vi "GUI_Bella_Control_Center_iP2.vi"() -> ()   [LabVIEW 2020]
uses:
  Shared/GUI_Template/GUI_master/tcp_new_data_event.ctl
  Shared/GUI_Template/GUI_master/tcp new data cluster.ctl
  GUI_TestStand/Fire button.ctl
  Device Drivers/DG645/subVIs/TriggerSource_TypDef.ctl
  <vilib>/Utility/config.llb/Write Key (I32).vi
  <vilib>/Platform/browser.llb/Open URL in Default Browser (string).vi
  <vilib>/Utility/config.llb/NI_LVConfig.lvlib
panel:
  in  "DPM intercept":dbl=94.0 format="%#_13g"
  in  "DPM Direction 3":bool=TRUE
  in  "Move SMF":bool=TRUE
  in  "DPM Direction":bool=TRUE
  in  "Move DPM":bool=TRUE
  in  "Position.Ch3::19":dbl caption="Target Microscope Z" min=0.0 max=100.0 format="%.3f"
  in  "GUIdevice 19":string="MCD-PL1-NewmarkDPMXZ"
  in  "Position.Axis 3::18":dbl caption="ESP6 focal spot mirror" min=0.0 max=100.0 format="%.3f"
  in  "Position.Axis 3::16":dbl caption="ESP5 Target Lateral" min=-200.0 max=200.0 format="%.3f"
  in  "Position.Axis 1::16":dbl caption="ESP5 Target Focus" min=-200.0 max=200.0 format="%.3f"
  in  "GUIdevice 18":string="MCD-PL1-NewmarkDPMXZ"
  in  "GUIdevice 16":string="MCD-PL1-NewmarkDPMXZ"
  in  "Position.Axis 1::14":dbl caption="Debris Shield" min=0.0 max=200.0 format="%.3f"
  in  "Position.Stage B::12":dbl caption="DPM Y" min=-100.0 max=105.0 format="%.3f"
  in  "Position.Stage C::11":dbl caption="DPM Z" min=-100.0 max=100.0 format="%.3f"
  in  "GUIdevice 14":string="MCD-PL1-NewmarkDPMXZ"
  in  "GUIdevice 12":string="MCD-PL1-NewmarkDPMXZ"
  in  "Position.Stage A::11":dbl caption="DPM X" min=-400.0 max=400.0 format="%.3f"
  in  "GUIdevice 11":string="MCD-PL1-NewmarkDPMXZ"
  out "got manpar ofi bool data":bool
  out "got manpar ofi data":bool
  out "set expt editor":bool
  in  "Delay.Ch D::10":dbl=-1.631e-06 caption="Delay D" min=-0.1 max=20.0 format="%.4f"
  in  "value6::42":dbl=0.006 caption="PostScanRate" min=0.1 max=1.0 format="%#_3f"
  in  "value5::42":dbl=0.006 caption="1BL-2BL-\nSplitter-Rpcnt" min=-9999999.0 max=9999999.0 format="%#_6p"
  in  "value6::43":bool=TRUE caption="GhostFoil-In"
  in  "value5::43":bool=TRUE caption="1BL-Energy\nMeter-In"
  in  "value4::43":bool=TRUE caption="2BLFoil-In"
  in  "value3::43":bool=TRUE caption="1BLFoil-In"
  in  "value2::43":bool=TRUE caption="ClunkerIn"
  out "CurrentStatus":string
  in  "MoveStage":bool
  in  "Position.Ch1::44":dbl caption="Current Position" min=0.0 max=150.0
  in  "GUIdevice 44":string="STAGE-LT-Megattenuator"
  in  "GUIdevice 43":string="MANPAR-BELLA-OFI-Boolean"
  in  "GUIdevice 42":string="MANPAR-BELLA-OFI"
  out "HPD2 to match HPD":dbl
  in  "Save \ncreenshots":bool
  out "error out":errorcluster
  out "HPD - focus":dbl
  in  "value1::42":dbl=230.0 caption="focus on HPD" min=-9999999.0 max=9999999.0
  in  "value0::43":bool=TRUE caption="SCS"
  in  "Thales.DIAG_CU_Output_Percent_1::37":dbl caption="Amp2 att (%)" min=1.0 max=100.0 step=500.0 format="%.2f"
  in  "GUIdevice 37":string="SVE-LT-Thales"
  in  "Scan":T1(ring)
  in  "LogTable":bool
  in  "New Google\nExpLog for new day?":bool=TRUE
  out "standard output":string
  in  "Create Log":bool caption="LogTable"
  in  "Position.Channel 5::31":T2(ring) caption="FROG foil"
  in  "Position.Channel 2::31":T2(ring) caption="Little Rick"
  in  "Step size 2":dbl=20.0 caption="Step size" min=-22.0 max=22.0
  in  "Position.Axis 4::33":dbl caption="Holy M V F4" min=-100000.0 max=100000.0 step=500.0
  in  "Position.Axis 3::33":dbl caption="Holy M H F3" min=-1000000.0 max=1000000.0 step=500.0
  in  "Position.Axis 2::33":dbl caption="Bessel M3 V F2" min=-100000.0 max=100000.0 step=500.0
  in  "Position.Axis 1::33":dbl caption="Bessel M3 H F1" min=-100000.0 max=100000.0 step=500.0
  in  "GUIdevice 33":string="MCD-PL1-picosOFI1"
  in  "GUIdevice 4":string="STAGE-PL1-Capstage1"
  in  "GUIdevice 31":string="1WIRE-BELLA-Flipper"
  in  "Amplitude.Ch GH::10":dbl=-1.631e-06 caption="Shot Shutter V" min=0.5 max=5.0 format="%.1f"
  in  "Rate (Hz)":dbl=0.3
  in  "Heater Alignment Directions":bool
  in  "Position.Axis 3::15":dbl caption="XY" min=-3.0 max=16.0 format="%.4f"
  in  "Position.Axis 2::15":dbl caption="Y" min=-3.0 max=17.0 format="%.4f"
  in  "Position.Axis 1::15":dbl caption="X" min=-3.0 max=13.0 format="%.4f"
  in  "GUIdevice 24":string="STAGE-HEAT-TL1"
  in  "Encoder position::23":dbl caption="position HPD2" min=0.0 max=600.0 format="%.1f"
  in  "position::3":dbl caption="position HPD" min=0.0 max=600.0 format="%.1f"
  in  "GUIdevice 23":string="STAGE-HPD-Far"
  in  "GUIdevice 22":string="MANPAR-BELLA-FireCont"
  in  "Allow Fire Continues":bool
  out "Fire continues Indicator":bool caption="firing"
  in  "Fire Button":T3=TRUE
  in  "Trigger.Source::10":T4 caption="SRS Trigger Mode"
  out "Absolute discharge timing":dbl caption="delay from pk" format="%#.3p"
  in  "Delay.Ch E::17":dbl caption="Timing box" min=-0.1 max=0.1 format="%.3p"
  in  "value0::22":bool caption="Fire continuosly"
  in  "GUIdevice 15":string="MCD-HEAT-ESP1"
  in  "GUIdevice 17":string="DDG-AA-SRS0"
  out "error IO 2":errorcluster
  out "tcp data event":T5
  in  "UDP error message":string
  in  "GUIdevice 13":string="DDG-AA-SRS2"
  in  "GUIdevice 2":string="MANPAR-BELLA-General"
  in  "GUIdevice 10":string="DDG-AA-ShotCntrl"
  in  "GUIdevice 1":string="HEX-PL1-1"
  in  "GUIdevice 3":string="STAGE-HPD-Tel"
  in  "Position.Axis 1::9":dbl caption="Comp1 Translation" min=-50.0 max=50.0 format="%.3f"
  in  "GUIdevice 9":string="STAGE-1BL-Compression"
  in  "stop":bool
  # "BELLA ip2 CONTROL CENTER"
  # "Scan"
  # "Safety"
  # "needs manpar-bella-ofi on\nMANPAR-BELLA-OFI-Boolean"
  # "Discharge timing (s)"
  # "1wire"
  # "DG"
  # "PICOS"
  # "Heater timing (s)"
  # "HPD Stage"
  # "Megattenuator Stage"
  # "Attenuate"
  # "OUT"
  # "IN"
  # "Compressor"
  # "Heater Alignment"
  # "Heat ESP0"
  # "Heat ESP1"
  # "Heat Pico"
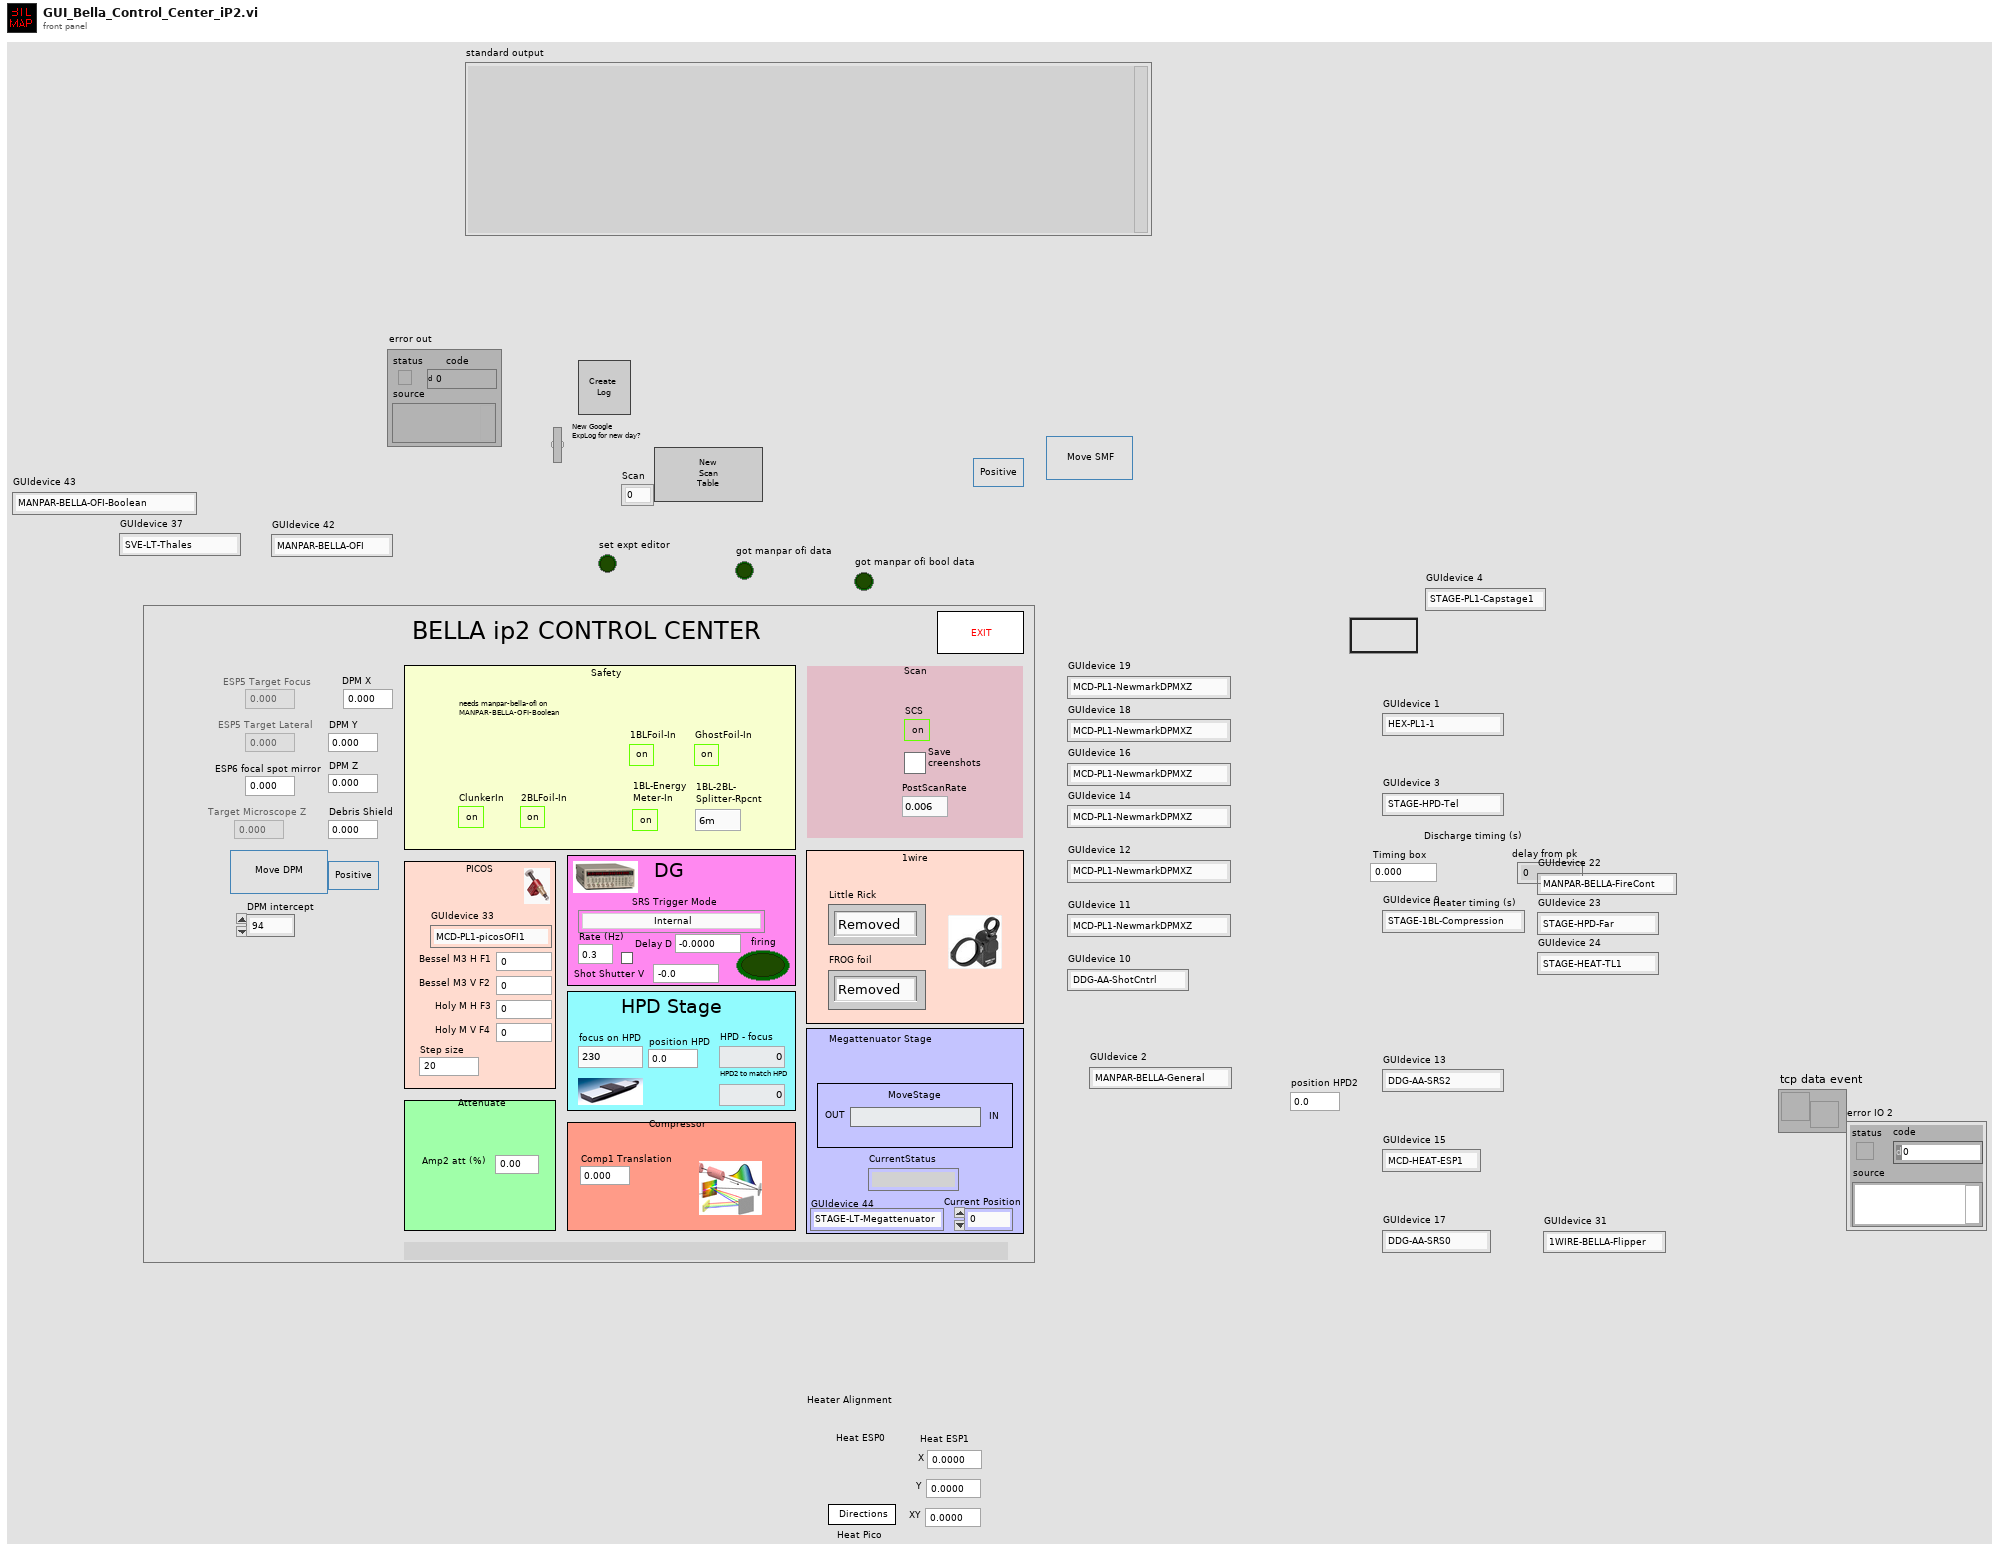
[diagram p1: front panel]
types:
  T1 = enum16{"0", "1", "2", "3", "4", "5", "6", "7", "8", "9", "10", "11", "12", "13", "14", "15", "16", "17", "18", "19", "20", "21", "22", "23", "24", "25", "26", "27", "28", "29", "30", "31", "32", "33", "34", "35", "36", "37", "38", "39", "40", "41", "42", "43", "44", "45", "46", "47", "48", "49", "50", "51", "52", "53", "54", "55", "56", "57", "58", "59", "60", "61", "62", "63", "64", "65", "66", "67", "68", "69", "70", "71", "72", "73", "74", "75", "76", "77", "78", "79", "81", "82", "83", "84", "85", "86", "87", "88", "89", "90", "91", "92", "93", "94", "95", "96", "97", "98", "99", ""}
  T2 = enum16{"Removed", "Inserted", "Unknown", "Moving"}
  T3 = typedef "Fire button.ctl" = bool
  T4 = typedef "TriggerSource_TypDef.ctl" = enum16{"Internal", "External rising edges", "External falling edges", "Single shot external rising edges", "Single shot external falling edges", "Single shot", "Line"}
  T5 = typedef "tcp_new_data_event.ctl" = refnum<user-event>
  T6 = typedef "tcp new data cluster.ctl" = cluster{"EventEnum":enum16{"new data", "connection status update"}, "Device name":string}
  T7 = enum8{"Enabled", "Disabled", "Disabled and Grayed Out"}
  T8 = enum32{"invalid app kind", "Development System", "Run Time System", "Student Edition", "Embedded LabVIEW", "Evaluation", "Custom"}
  T9 = enum32{"Invalid", "Standard", "Closed", "Hidden", "Minimized", "Maximized"}
  T10 = typedef "imagedata.ctl" = cluster{"image type":i32, "image depth":i32, "image":u8[], "mask":u8[], "colors":u32[], "Rectangle":cluster{"left":i16, "top":i16, "right":i16, "bottom":i16}}
  T11 = typedef "NI_LVConfig.lvlib/Config Data RefNum.ctl" = refnum<k1>
  T12 = cluster{"Core":cluster{"Current VI Reference":refnum<vi>, "Close Panel on Exit?":bool}, "Heater timing offset":dbl, "Discharge timing offset":dbl, "Jet trigger":bool, "Tik1":u32, "Tik2":u32, "Fire Continues Allowed":bool}
  T13 = cluster{"Current VI Reference":refnum<vi>, "Close Panel on Exit?":bool}
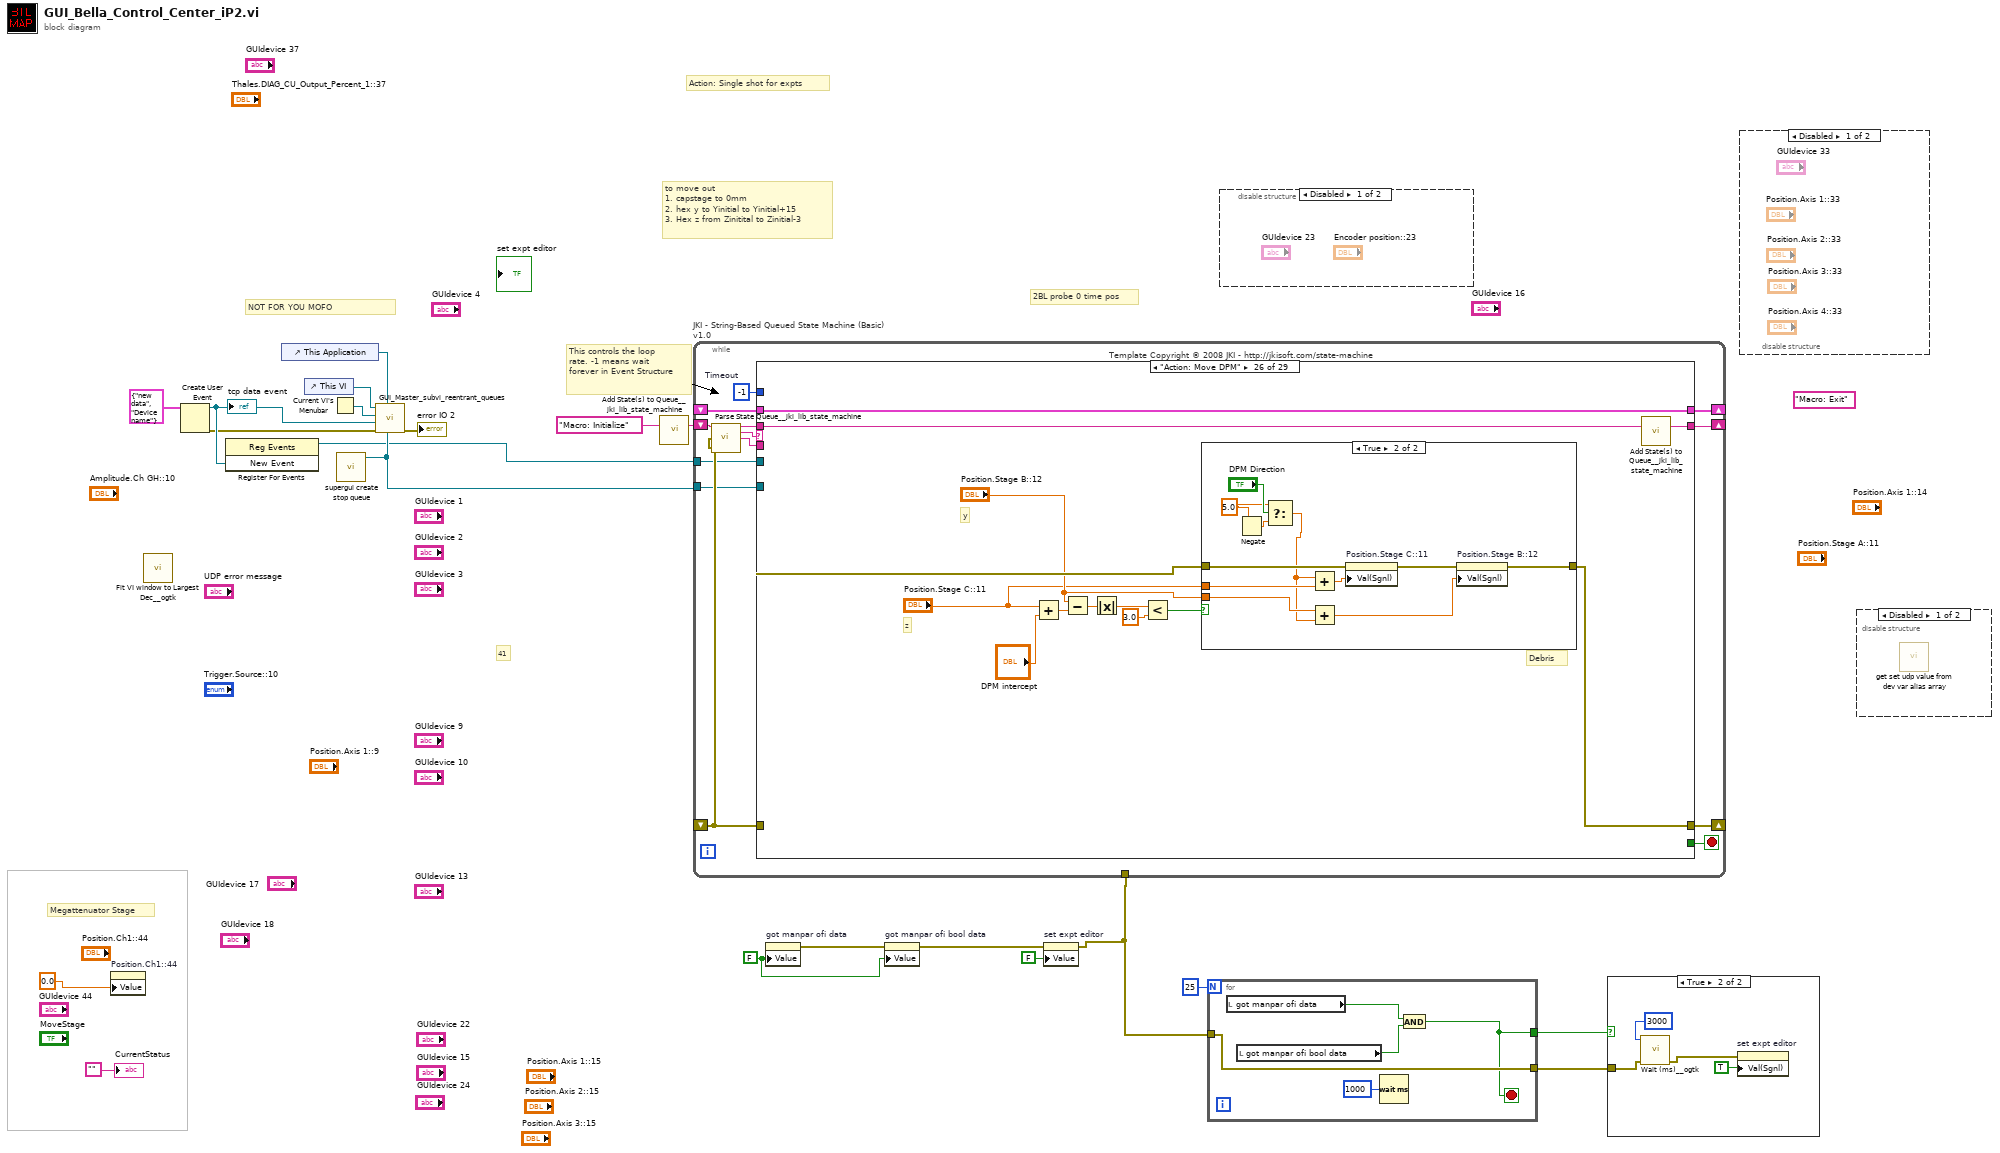
[diagram p0: block diagram]
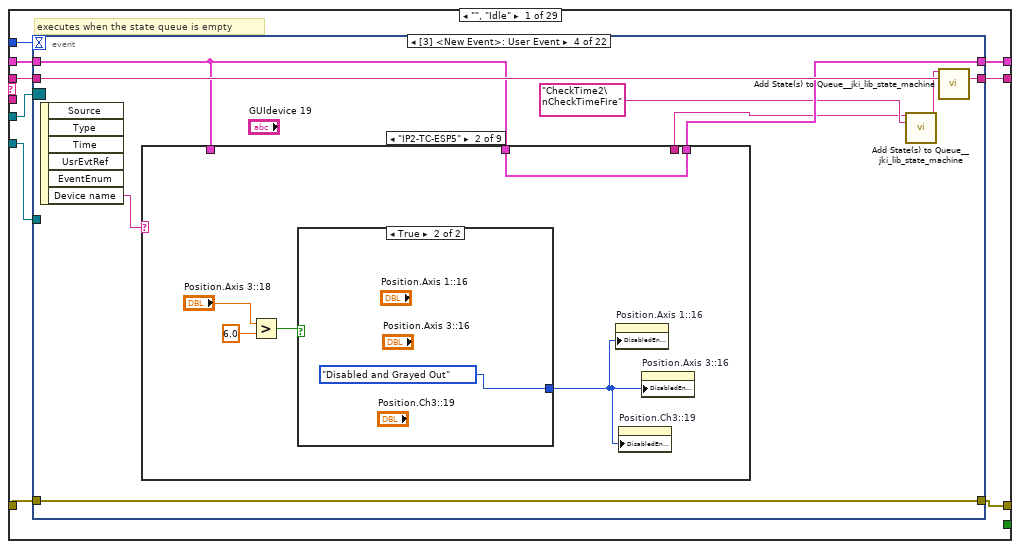
[diagram p6: hidden frame]
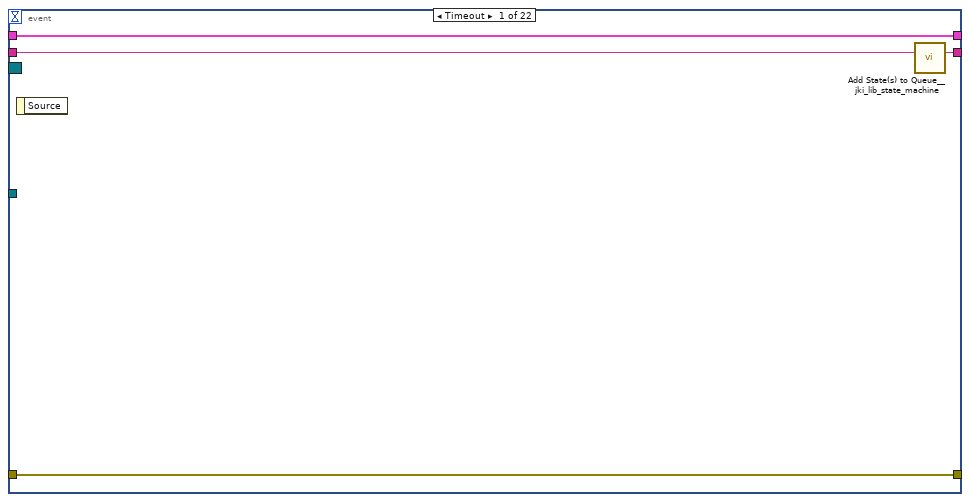
[diagram p7: hidden frame]
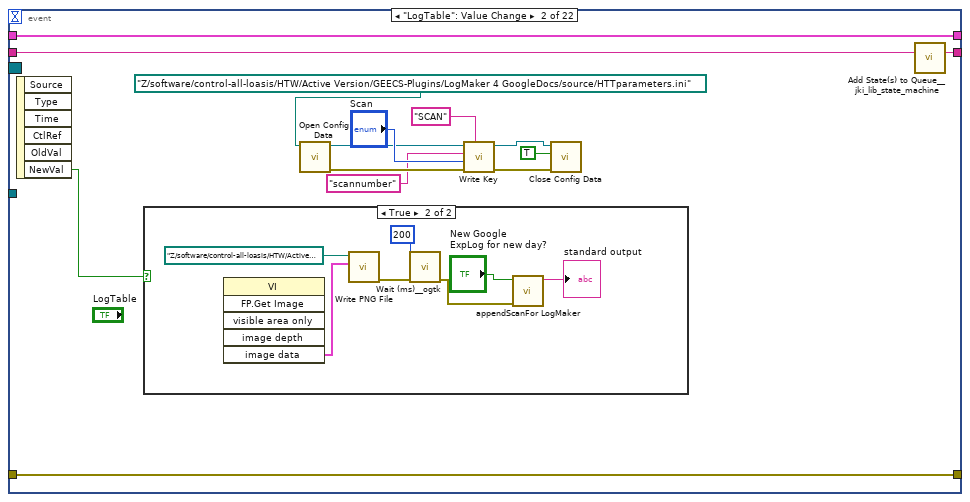
[diagram p8: hidden frame]
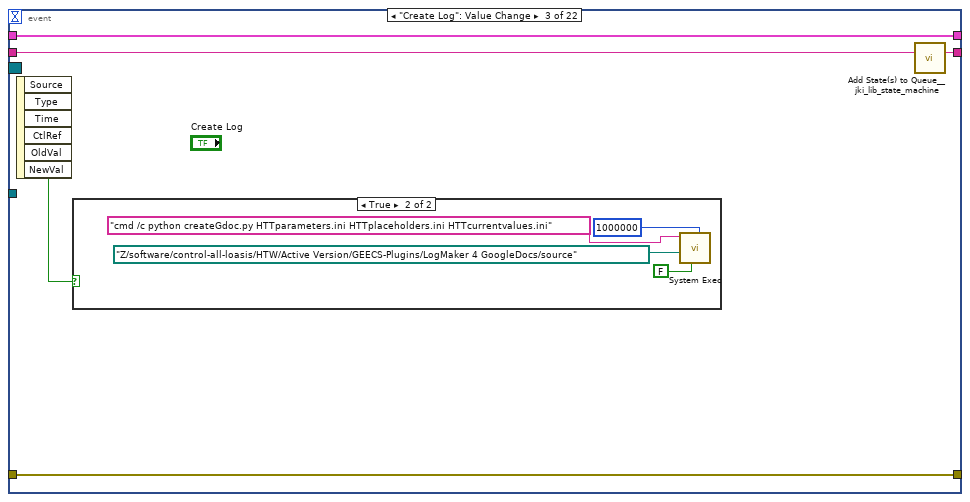
[diagram p10: hidden frame]
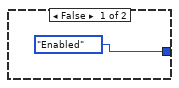
[diagram p13: hidden frame]
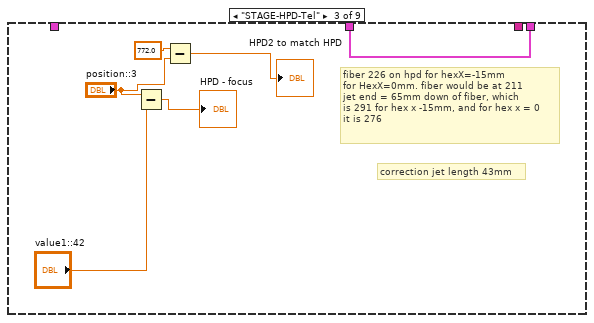
[diagram p14: hidden frame]
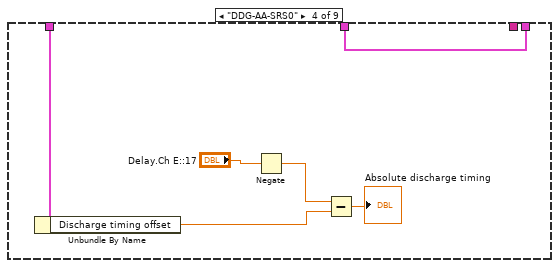
[diagram p15: hidden frame]
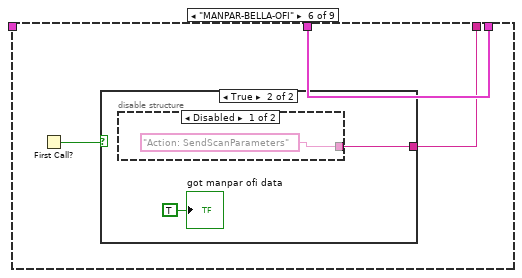
[diagram p17: hidden frame]
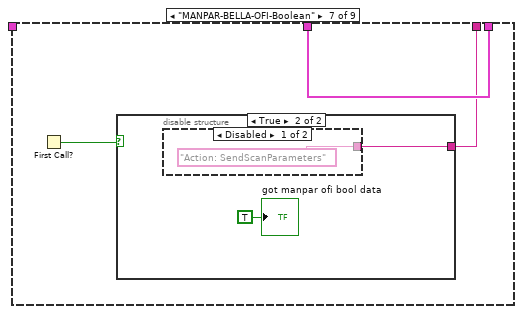
[diagram p20: hidden frame]
diagram:
  w5 = FALSE ("got manpar ofi data")
  (unwired) "Macro: Exit"
  # "41"
  # "Megattenuator Stage"
  # "2BL probe 0 time pos"
  # "Action: Single shot for expts"
  # "to move out\n1. capstage to 0mm\n2. hex y to Yinitial to Yinitial+15\n3. Hex z from Zinitital to Zinitial-3"
  # "This controls the loop rate. -1 means wait forever in Event Structure"
  # "NOT FOR YOU MOFO"
  n1 = property on="Position.Ch1::44" class="DigNum (strict)"("Value"=0.0 ("Position.Ch1::44")) -> ()  [unwired: 2 in, 2 out]
  n2 = call <userlib>:"Fit VI window to Largest Dec__ogtk.vi"() -> ()  [unwired: 6 in, 2 out]
  n3 = Create User Event(user event datatype=T6 {"EventEnum"=enum."new data", "Device name"="Device name"} ("New Event")) -> (user event=w20:refnum<user-event>, error out=w19:errorcluster)  [unwired: 1 in]
  "tcp data event" <- w20
  n4 = register-events(w20) -> (reference out=w11:refnum<event-registration>)  [unwired: 2 in, 1 out]
  n5 = control-ref of="This Application"() -> (w21:refnum<vi>)
  n6 = control-ref of="This VI"() -> (w15:refnum<vi>)
  n7 = Current VI's Menubar() -> (w17:refnum<k9>)
  n8 = call "supergui create stop queue.vi"() -> ("STOP Queue out"=w12:refnum<queue>)  [unwired: 11 in]
  n9 = call "GUI_Master_subvi_reentrant_queues.vi"("STOP Queue in"=w12, "This Application"=w21, "error in (no error)"=w19, "tcp data event"=w20, "Caller menu reference"=w17, "Caller VI ref"=w15) -> ("error out"=→"error IO 2":errorcluster)  [unwired: 5 in]
  n10 = call <vilib>:"Add State(s) to Queue__jki_lib_state_machine.vi"("State(s) in (\"\")"="Macro: Initialize") -> ("States Out"=w13:string)  [unwired: 14 in]
  n11 = property on="got manpar ofi data" class="Bool (strict)"("Value"=w5) -> (error out=w6:errorcluster)  [unwired: 2 in, 1 out]
  n12 = property on="got manpar ofi bool data" class="Bool (strict)"(error in=w6, "Value"=w5) -> (error out=w7:errorcluster)  [unwired: 1 in, 1 out]
  n13 = property on="set expt editor" class="Bool (strict)"(error in=w7, "Value"=FALSE ("set expt editor")) -> (error out=w4:errorcluster)  [unwired: 1 in, 1 out]
  n14 = while "JKI - String-Based Queued State Machine (Basic) v1.0" {
    shift-right: [w27] -> _
    shift-left: _ -> [w26]
    shift-right: [w30] -> _
    shift-left: _ -> [w24]
    shift-right: [w29] -> _
    shift-left: w13 -> [w31]
    tunnel: w11 -> [w23]
    tunnel: w12 -> [w22]
    tunnel: w4 -> [_]
    stop <- w28 stop-if-true
    w25 = -1  # Timeout
    # "Template Copyright © 2008 JKI - http://jkisoft.com/state-machine"
    n15 = call <vilib>:"Parse State Queue__jki_lib_state_machine.vi"("State Queue"=w31, "Error In (no error)"=w24) -> ("Remaining States"=w33:string, "Current State"=w34:string, "Arguments"=w32:string)  [unwired: 11 in]
    n16 = case shown="\"Action: Move DPM\"" w34 {
      selector: w34 -> [_ _ w296 _ _ _ _ _ _ _ _ _ _ _ _ _ _ _ _ _ _ _ _ _ _ _ _ _ _]
      tunnel: w33 -> [w43 w295 w300 w318 w324 w329 w333 w344 w350 w354 w358 w364 w375 w401 w406 w419 w423 w429 w438 w475 w486 w498 w510 w517 w521 w534 w550 w558 w565]
      tunnel: w32 -> [_ _ _ _ _ _ _ _ _ _ _ w359 w369 _ _ _ _ _ _ _ _ _ _ _ _ _ _ _ _]
      tunnel: w26 -> [w41 w292 w298 w309 w321 w327 w330 _ w345 w351 w356 w362 w371 w398 w403 w416 w420 w426 w435 w463 w482 w492 w507 w515 w519 w532 w547 w555 w562]
      tunnel: [w40 w293 w302 w315 errorcluster {"status"=FALSE, "code"=0, "source"=""} ("error out") w326 w331 w341 w346 w352 w355 w360 w372 w399 w404 w417 w421 w427 w436 w473 w480 w487 w508 w514 w518 w524 w548 w556 w563] -> w30
      tunnel: w24 -> [w39 w293 w301 w315 w320 w326 w331 w341 w347 w352 w355 w361 w373 w399 w404 w417 w421 w427 w436 w473 w484 w488 w508 w514 w518 w525 w548 w556 w563]
      tunnel: [w42 w294 w299 w317 w323 w328 w332 w343 w349 w353 w357 w363 w374 w400 w405 w418 w422 w428 w437 w474 w485 w497 w509 w516 w520 w533 w549 w557 w564] -> w29
      tunnel: [_ _ _ _ _ TRUE _ _ _ _ _ _ _ _ _ _ _ _ _ _ _ _ _ _ _ _ _ _ _] -> w28
      tunnel: [w35 w292 w298 w316 w321 w327 w330 w342 w345 w351 w356 w362 w371 w398 w403 w416 w420 w426 w435 w472 w482 w491 w506 w515 w519 w532 w547 w555 w562] -> w27
      tunnel: w25 -> [w38 _ _ _ _ _ _ _ _ _ _ _ _ _ _ _ _ _ _ _ _ _ _ _ _ _ _ _ _]
      tunnel: w23 -> [w37 _ _ _ _ _ _ _ _ _ _ _ _ _ _ _ _ _ _ _ _ _ _ _ _ _ _ _ _]
      tunnel: w22 -> [w36 _ _ _ _ _ _ _ _ _ _ _ _ _ _ w408 _ _ _ _ _ _ _ _ _ _ _ _ _]
      frame "", "Idle" {
        # "executes when the state queue is empty"
        n17 = event shown="[3] <New Event>: User Event" {
          selector: w37 -> [_ _ _ _ _ _ _ _ _ _ _ _ _ _ _ _ _ _ _ _ _ _]
          dyn-events: _ -> [_ _ _ _ _ _ _ _ _ _ _ _ _ _ _ _ _ _ _ _ _ _]
          timeout: w38 -> [_ _ _ _ _ _ _ _ _ _ _ _ _ _ _ _ _ _ _ _ _ _]
          tunnel: w43 -> [w47 w61 w73 w86 w129 w131 w136 w141 w146 w156 w166 w176 w186 w196 w205 w213 w222 w246 w256 w263 w265 w291]
          tunnel: [w46 w60 w72 w85 w128 w132 w137 w142 w147 w157 w167 w177 w187 w197 w206 w213 w221 w244 w256 w263 w264 w290] -> w42
          tunnel: w41 -> [w44 w58 w70 w82 w126 w134 w139 w144 w149 w159 w169 w179 w189 w199 w208 w212 w224 w248 w257 w262 w272 w288]
          tunnel: [w45 w59 w71 w84 w127 w133 w138 w143 w148 w158 w168 w178 w188 w198 w207 w210 w227 w247 w255 w261 w271 w289] -> w40
          tunnel: w39 -> [w45 w59 w71 w84 w127 w133 w138 w143 w148 w158 w168 w178 w188 w198 w207 w211 w226 w247 w255 w261 w271 w289]
          tunnel: [w44 w58 w70 w81 w126 w134 w139 w144 w149 w159 w169 w179 w189 w199 w208 w212 w225 w248 w257 w262 w272 w288] -> w35
          tunnel: w36 -> [_ _ _ _ _ _ _ _ _ _ _ _ _ _ _ _ _ _ _ _ _ _]
          event Timeout {
            n18 = event-data() -> ()  [unwired: 1 in, 1 out]
            n19 = call <vilib>:"Add State(s) to Queue__jki_lib_state_machine.vi"("State(s) in (\"\")"=w47) -> ("States Out"=w46:string)  [unwired: 14 in]
          }
          event "LogTable": Value Change {
            n20 = event-data() -> ("NewVal"=w48:bool)  [unwired: 1 in, 5 out]
            n21 = case shown="True" w48 {
              frame False {
              }
              frame True {
                n22 = invoke class="VI" method="FP.Get Image"() -> ("image data"=w68:T10)  [unwired: 6 in, 5 out]
                n23 = call <vilib>:"Write PNG File.vi"("image data"=w68, "path to PNG file"=path "Z:/software/control-all-loasis/HTW/Active Version/GEECS-Plugins/LogMaker 4 GoogleDocs/source/frontpanel.png" ("report file path")) -> ("error out"=w63:errorcluster)  [unwired: 8 in, 1 out]
                n24 = call <userlib>:"Wait (ms)__ogtk.vi"("error in (no error)"=w63, "milliseconds to wait"=u32 200 ("millisecond timer value")) -> ("error out"=w62:errorcluster)  [unwired: 8 in, 1 out]
                n25 = call "appendScanFor LogMaker.vi"("error in (no error)"=w62, "New Google\nExpLog for new day?"="New Google\nExpLog for new day?") -> ("standard output"=→"standard output":string)  [unwired: 9 in]
              }
            }
            n26 = call <vilib>:"Open Config Data.vi"("configuration file path"=path "Z:/software/control-all-loasis/HTW/Active Version/GEECS-Plugins/LogMaker 4 GoogleDocs/source/HTTparameters.ini") -> ("error out"=w55:errorcluster, "refnum"=w53:T11)  [unwired: 8 in, 1 out]
            n27 = call-poly <vilib>:"Write Key.vi"("section"="SCAN", "error in (no error)"=w55, "value"="Scan", "key"="scannumber", "refnum"=w53) -> ("error out"=w56:errorcluster, "refnum out"=w54:T11)  [unwired: 4 in, 1 out]
            n28 = call <vilib>:"Close Config Data.vi"("error in (no error)"=w56, "write file if changed (T)"=TRUE, "refnum"=w54) -> ()  [unwired: 7 in, 2 out]
            n29 = call <vilib>:"Add State(s) to Queue__jki_lib_state_machine.vi"("State(s) in (\"\")"=w61) -> ("States Out"=w60:string)  [unwired: 14 in]
          }
          event "Create Log": Value Change {
            n30 = event-data() -> ("NewVal"=w69:bool)  [unwired: 1 in, 5 out]
            n31 = case shown="True" w69 {
              frame False {
              }
              frame True {
                n32 = call <vilib>:"System Exec.vi"("expected output size  (4096)"=u32 1000000, "run minimized? (F)"=FALSE, "working directory"=path "Z:/software/control-all-loasis/HTW/Active Version/GEECS-Plugins/LogMaker 4 GoogleDocs/source", "command line"="cmd /c python createGdoc.py HTTparameters.ini HTTplaceholders.ini HTTcurrentvalues.ini") -> ()  [unwired: 4 in, 4 out]
              }
            }
            n33 = call <vilib>:"Add State(s) to Queue__jki_lib_state_machine.vi"("State(s) in (\"\")"=w73) -> ("States Out"=w72:string)  [unwired: 14 in]
          }
          event User Event {
            n34 = event-data() -> ("Device name"=w83:string)  [unwired: 1 in, 5 out]
            n35 = case shown="\"IP2-TC-ESP5\"" w83 {
              tunnel: w82 -> [_ _ _ w103 _ _ _ _ _]
              tunnel: w82 -> [w87 w92 w100 w101 w107 w110 w116 w123 w124]
              tunnel: [w87 w92 w100 w101 w107 w110 w116 w123 w124] -> w81
              tunnel: [_ _ _ _ _ w109 w115 "Check Megattenuator Stage Status" ("State(s) in Front (\"\")") _] -> w78
              frame "False", Default {
              }
              frame "IP2-TC-ESP5" {
                n36 = Greater?(x="Position.Axis 3::18", y=6.0) -> (0:w89:bool)
                n37 = case shown="True" w89 {
                  tunnel: [T7."Enabled" ("Disabled") T7."Disabled and Grayed Out" ("Disabled")] -> w88
                  frame False {
                  }
                  frame True {
                  }
                }
                n38 = property on="Position.Axis 1::16" class="DigNum (strict)"("DisabledEnum"=w88) -> ()  [unwired: 2 in, 2 out]
                n39 = property on="Position.Ch3::19" class="DigNum (strict)"("DisabledEnum"=w88) -> ()  [unwired: 2 in, 2 out]
                n40 = property on="Position.Axis 3::16" class="DigNum (strict)"("DisabledEnum"=w88) -> ()  [unwired: 2 in, 2 out]
              }
              frame "STAGE-HPD-Tel" {
                # "correction jet length 43mm"
                # "fiber 226 on hpd for hexX=-15mm\nfor HexX=0mm. fiber would be at 211\njet end = 65mm down of fiber, which\nis 291 for hex x -15mm, and for hex x = 0\nit is 276"
                n41 = Subtract(x="position::3", y="value1::42") -> (x-y=→"HPD - focus":dbl)
                n42 = Subtract(x=772.0 ("y"), y="position::3") -> (x-y=→"HPD2 to match HPD":dbl)
              }
              frame "DDG-AA-SRS0" {
                n43 = Unbundle By Name(w103) -> ("Discharge timing offset"=w102:dbl)
                n44 = Negate(x="Delay.Ch E::17") -> (-x=w104:dbl)
                n45 = Subtract(x=w104, y=w102) -> (x-y=→"Absolute discharge timing":dbl)
              }
              frame "STAGE-2BL-ProbeDelay" {
              }
              frame "MANPAR-BELLA-OFI" {
                n46 = First Call?() -> (First Call?: T/F=w108:bool)
                n47 = case shown="True" w108 {
                  tunnel: [_ w112] -> w109
                  frame False {
                  }
                  frame True {
                    n48 = disable-structure shown="Disabled" {
                      disable-tunnel: ["Action: SendScanParameters" ("State(s) in Front (\"\")") _] -> w112
                      frame Disabled {
                      }
                      frame Enabled {
                      }
                    }
                    "got manpar ofi data" <- TRUE ("got manpar ofi data")
                  }
                }
              }
              frame "MANPAR-BELLA-OFI-Boolean" {
                n49 = First Call?() -> (First Call?: T/F=w114:bool)
                n50 = case shown="True" w114 {
                  tunnel: [_ w118] -> w115
                  frame False {
                  }
                  frame True {
                    n51 = disable-structure shown="Disabled" {
                      disable-tunnel: ["Action: SendScanParameters" ("State(s) in Front (\"\")") _] -> w118
                      frame Disabled {
                      }
                      frame Enabled {
                      }
                    }
                    "got manpar ofi bool data" <- TRUE ("got manpar ofi bool data")
                  }
                }
              }
              frame "STAGE-LT-Megattenuator" {
                n52 = property on="Position.Ch1::44" class="DigNum (strict)"() -> ("Caption.FontStrike"=w120:bool)  [unwired: 2 in, 2 out]
                n53 = Not(x=w120) -> (.not. x?=w121:bool)
                n54 = property on="MoveStage" class="Bool (strict)"("Visible"=w121) -> ()  [unwired: 2 in, 2 out]
                n55 = property on="CurrentStatus" class="Str"("Visible"=w121) -> ()  [unwired: 2 in, 2 out]
              }
              frame "1WIRE-BELLA-Flipper" {
              }
            }
            n56 = call <vilib>:"Add State(s) to Queue__jki_lib_state_machine.vi"("State(s) in Front (\"\")"=w78, "State(s) in (\"\")"="CheckTime2\nCheckTimeFire" ("State(s) in Front (\"\")")) -> ("States Out"=w79:string)  [unwired: 13 in]
            n57 = call <vilib>:"Add State(s) to Queue__jki_lib_state_machine.vi"("State(s) in Front (\"\")"=w79, "State(s) in (\"\")"=w86) -> ("States Out"=w85:string)  [unwired: 13 in]
          }
          event "stop": Value Change {
            # "Exit Button Value Change (pressed) Event\n(this executes Macro: Exit to terminate the VI)"
            n58 = event-data() -> ()  [unwired: 1 in, 6 out]
            n59 = call <vilib>:"Add State(s) to Queue__jki_lib_state_machine.vi"("State(s) in Front (\"\")"="Macro: Exit", "State(s) in (\"\")"=w129) -> ("States Out"=w128:string)  [unwired: 13 in]
          }
          event Value Change {
            n60 = event-data() -> ()  [unwired: 1 in, 6 out]
            n61 = call <vilib>:"Add State(s) to Queue__jki_lib_state_machine.vi"("State(s) in Front (\"\")"="Action: Fire" ("State(s) in Front (\"\")"), "State(s) in (\"\")"=w131) -> ("States Out"=w132:string)  [unwired: 13 in]
          }
          event "Move DPM": Value Change {
            n62 = event-data() -> ()  [unwired: 1 in, 6 out]
            n63 = call <vilib>:"Add State(s) to Queue__jki_lib_state_machine.vi"("State(s) in Front (\"\")"="Action: Move DPM" ("State(s) in Front (\"\")"), "State(s) in (\"\")"=w136) -> ("States Out"=w137:string)  [unwired: 13 in]
          }
          event "Move SMF": Value Change {
            n64 = event-data() -> ()  [unwired: 1 in, 6 out]
            n65 = call <vilib>:"Add State(s) to Queue__jki_lib_state_machine.vi"("State(s) in Front (\"\")"="Action: Move SMF" ("State(s) in Front (\"\")"), "State(s) in (\"\")"=w141) -> ("States Out"=w142:string)  [unwired: 13 in]
          }
          event "value0::43", "value6::42": Value Change {
            n66 = event-data() -> ()  [unwired: 1 in, 6 out]
            n67 = call <vilib>:"Add State(s) to Queue__jki_lib_state_machine.vi"("State(s) in Front (\"\")"="Action: SendScanParameters" ("State(s) in Front (\"\")"), "State(s) in (\"\")"=w146) -> ("States Out"=w147:string)  [unwired: 13 in]
          }
          event "value2::43": Value Change {
            n68 = event-data() -> ()  [unwired: 1 in, 6 out]
            n69 = local read "GUIdevice 43"() -> (w150:string)
            n70 = Select(t="on", s="value2::43", f="off") -> (s? t:f=w155:string)
            n71 = call "DefaultValue_Variable_MC.vi"("Variable In"="value2", "Default Value"=w155, "Device In"=w150) -> ()  [unwired: 1 in]
            n72 = call <vilib>:"Add State(s) to Queue__jki_lib_state_machine.vi"("State(s) in (\"\")"=w156) -> ("States Out"=w157:string)  [unwired: 14 in]
          }
          event "value3::43": Value Change {
            n73 = event-data() -> ()  [unwired: 1 in, 6 out]
            n74 = local read "GUIdevice 43"() -> (w161:string)
            n75 = Select(t="on", s="value3::43", f="off") -> (s? t:f=w165:string)
            n76 = call "DefaultValue_Variable_MC.vi"("Variable In"="value3", "Default Value"=w165, "Device In"=w161) -> ()  [unwired: 1 in]
            n77 = call <vilib>:"Add State(s) to Queue__jki_lib_state_machine.vi"("State(s) in (\"\")"=w166) -> ("States Out"=w167:string)  [unwired: 14 in]
          }
          event "value4::43": Value Change {
            n78 = event-data() -> ()  [unwired: 1 in, 6 out]
            n79 = local read "GUIdevice 43"() -> (w171:string)
            n80 = Select(t="on", s="value4::43", f="off") -> (s? t:f=w175:string)
            n81 = call "DefaultValue_Variable_MC.vi"("Variable In"="value4", "Default Value"=w175, "Device In"=w171) -> ()  [unwired: 1 in]
            n82 = call <vilib>:"Add State(s) to Queue__jki_lib_state_machine.vi"("State(s) in (\"\")"=w176) -> ("States Out"=w177:string)  [unwired: 14 in]
          }
          event "value5::43": Value Change {
            n83 = event-data() -> ()  [unwired: 1 in, 6 out]
            n84 = local read "GUIdevice 43"() -> (w181:string)
            n85 = Select(t="on", s="value5::43", f="off") -> (s? t:f=w185:string)
            n86 = call "DefaultValue_Variable_MC.vi"("Variable In"="value5", "Default Value"=w185, "Device In"=w181) -> ()  [unwired: 1 in]
            n87 = call <vilib>:"Add State(s) to Queue__jki_lib_state_machine.vi"("State(s) in (\"\")"=w186) -> ("States Out"=w187:string)  [unwired: 14 in]
          }
          event "value6::43": Value Change {
            n88 = event-data() -> ()  [unwired: 1 in, 6 out]
            n89 = local read "GUIdevice 43"() -> (w191:string)
            n90 = Select(t="on", s="value6::43", f="off") -> (s? t:f=w195:string)
            n91 = call "DefaultValue_Variable_MC.vi"("Variable In"="value6", "Default Value"=w195, "Device In"=w191) -> ()  [unwired: 1 in]
            n92 = call <vilib>:"Add State(s) to Queue__jki_lib_state_machine.vi"("State(s) in (\"\")"=w196) -> ("States Out"=w197:string)  [unwired: 14 in]
          }
          event "value5::42": Value Change {
            n93 = event-data() -> ()  [unwired: 1 in, 6 out]
            n94 = Number To Fractional String(number="value5::42", precision (6)=i16 4) -> (F-format string=w201:string)  [unwired: 2 in]
            n95 = call "DefaultValue_Variable_MC.vi"("Variable In"="value5", "Default Value"=w201, "Device In"="GUIdevice 42") -> ()  [unwired: 1 in]
            n96 = call <vilib>:"Add State(s) to Queue__jki_lib_state_machine.vi"("State(s) in (\"\")"=w205) -> ("States Out"=w206:string)  [unwired: 14 in]
          }
          event "Heater Alignment Directions": Value Change {
            n97 = event-data() -> ()  [unwired: 1 in, 6 out]
            n98 = case shown="True" "Heater Alignment Directions" {
              tunnel: w211 -> [w214 w217]
              tunnel: [w214 w216] -> w210
              frame False {
              }
              frame True {
                n99 = call-poly <vilib>:"Open URL in Default Browser.vi"("error in (no error)"=w217, "URL"="https://docs.google.com/document/d/1RMZp6W8Kkog2nkTymSjyZ2bh9D7Vo4bxhvGgn3Ut4KE/edit") -> ("error out"=w216:errorcluster)  [unwired: 4 in, 1 out]
              }
            }
          }
          event "Allow Fire Continues": Value Change {
            n100 = event-data() -> ()  [unwired: 1 in, 6 out]
            n101 = Unbundle By Name(w224) -> ("Fire Continues Allowed"=w223:bool)
            n102 = case shown="True" "Allow Fire Continues" {
              tunnel: [w228 w235] -> w227
              tunnel: "Allow Fire Continues" -> [_ w234]
              tunnel: w226 -> [w228 w233]
              tunnel: w223 -> [w229 w232]
              tunnel: [w229 w230] -> w219
              tunnel: [_ "Initilize Fire Continues" ("State(s) in Front (\"\")")] -> w218
              frame False {
              }
              frame True {
                n103 = case shown="False" w232 {
                  tunnel: [w241 w242] -> w235
                  tunnel: w234 -> [w240 _]
                  tunnel: w233 -> [w239 w242]
                  tunnel: [w236 FALSE] -> w230
                  frame False {
                    n104 = call "Password"("Enable"=w240, "error in (no error)"=w239) -> ("Password"=w238:string, "error out"=w241:errorcluster)  [unwired: 15 in, 1 out]
                    n105 = Equal?(x=w238, y="fire") -> (x = y?=w236:bool)
                  }
                  frame True {
                  }
                }
              }
            }
            n106 = Bundle By Name(cluster=w224, "Fire Continues Allowed"=w219) -> (w225:T12)
            n107 = call <vilib>:"Add State(s) to Queue__jki_lib_state_machine.vi"("State(s) in Front (\"\")"=w218, "State(s) in (\"\")"=w222) -> ("States Out"=w221:string)  [unwired: 13 in]
          }
          event "set expt editor": Value Change {
            n108 = event-data() -> ()  [unwired: 1 in, 6 out]
            n109 = call <vilib>:"Add State(s) to Queue__jki_lib_state_machine.vi"("State(s) in Front (\"\")"="Action: SendScanParameters" ("State(s) in Front (\"\")"), "State(s) in (\"\")"=w246) -> ("States Out"=w244:string)  [unwired: 13 in]
          }
          event "Step size 2": Value Change {
            n110 = event-data() -> ("NewVal"=w249:dbl)  [unwired: 1 in, 5 out]
            n111 = control-ref of="Position.Axis 1::33"() -> (w254:refnum<vi>)
            n112 = control-ref of="Position.Axis 2::33"() -> (w253:refnum<vi>)
            n113 = control-ref of="Position.Axis 4::33"() -> (w251:refnum<vi>)
            n114 = control-ref of="Position.Axis 3::33"() -> (w252:refnum<vi>)
            n115 = Build Array(w254, w253, w252, w251) -> (w250:refnum<vi>[])
            n116 = for {
              tunnel: w250 -> [w259] mode=indexing
              tunnel: w249 -> [w258]
              n117 = property on="Property Node" class="DigNum (strict)"(reference=w259, "Increment"=w258) -> ()  [unwired: 1 in, 2 out]
            }
          }
          event Value Change {
            n118 = event-data() -> ()  [unwired: 1 in, 6 out]
            n119 = property on="value0::22" class="Bool (strict)"("Val(Sgnl)"=FALSE) -> ()  [unwired: 2 in, 2 out]
          }
          event "MoveStage": Value Change {
            n120 = event-data() -> ("OldVal"=w267:bool, "NewVal"=w270:bool)  [unwired: 1 in, 4 out]
            n121 = flat-sequence {
              tunnel: w270 -> [w277]
              tunnel: [w277] -> w269
              tunnel: [w274] -> w268
              tunnel: w267 -> [w273]
              tunnel: [w273] -> w266
              tunnel: w269 -> [w280]
              tunnel: w268 -> [w279]
              tunnel: w266 -> [w278]
              frame #0 {
                n122 = call "PasswordPrompt.vi"() -> ("Please enter password below 2"=w276:string)  [unwired: 11 in]
                n123 = Equal?(x=w276, y="l0dat&srv!") -> (x = y?=w274:bool)
              }
              frame #1 {
                n124 = case shown="True" w279 {
                  tunnel: w280 -> [_ w283]
                  tunnel: w278 -> [w281 _]
                  frame False {
                    n125 = call "Display Message to User"("Message"="Wrong Password") -> ()  [unwired: 9 in, 2 out]
                    n126 = property on="MoveStage" class="Bool (strict)"("Value"=w281) -> ()  [unwired: 2 in, 2 out]
                  }
                  frame True {
                    n127 = case shown="True" w283 {
                      frame False {
                        n128 = property on="Position.Ch1::44" class="DigNum (strict)"("Val(Sgnl)"=150.0 ("Value (Signaling)")) -> ()  [unwired: 2 in, 2 out]
                      }
                      frame True {
                        n129 = property on="Position.Ch1::44" class="DigNum (strict)"("Val(Sgnl)"=0.5 ("Value (Signaling)")) -> ()  [unwired: 2 in, 2 out]
                      }
                    }
                    n130 = property on="MoveStage" class="Bool (strict)"("Value"=w283) -> ()  [unwired: 2 in, 2 out]
                  }
                }
              }
            }
            n131 = call <vilib>:"Add State(s) to Queue__jki_lib_state_machine.vi"("State(s) in (\"\")"=w265) -> ("States Out"=w264:string)  [unwired: 14 in]
          }
          event Panel Close? {
            # "Discard the event because we'll close the front panel ourselves in Macro: Exit"
            # "Close Panel button (pressed) Event\n(this executes Macro: Exit to terminate the VI)"
            n132 = event-data() -> ()  [unwired: 1 in, 1 out]
            n133 = event-data("Discard?"=TRUE) -> ()  [unwired: 1 in, 1 out]
            n134 = call <vilib>:"Add State(s) to Queue__jki_lib_state_machine.vi"("State(s) in Front (\"\")"="Macro: Exit", "State(s) in (\"\")"=w291) -> ("States Out"=w290:string)  [unwired: 13 in]
          }
        }
      }
      frame "---------- Core ----------" {
        # "Do not put any code in this frame.\n(it is a separator no-op)"
        n135 = call <vilib>:"Add State(s) to Queue__jki_lib_state_machine.vi"("State(s) in (\"\")"=w295) -> ("States Out"=w294:string)  [unwired: 14 in]
      }
      frame Default {
        w305 = 42 items=["No error", "Argument error", "Memory is full", "Out of zone", "End of file", "File already open", "Generic file I/O error", "File not found", "File permission error", "Disk is full", "Duplicate path", "Too many files open", "System feature not enabled", "Resource file not found", "Cannot add resource", "Resource not found", "Image not found", "Image memory error", "Pen does not exist", "Config type invalid", "Config token not found", "Config parse error", "Config memory error", "Bad external code format", "Bad external code offset", "External code not present", "Null window", "Destroy window error", "Null menu", "Print aborted", "Bad print record", "Print driver error", "Windows error during printing", "Memory error during printing", "Print dialog error", "Generic print error", "Invalid device refnum", "Device not found", "Device parameter error", "Device unit error", "Cannot open device", "Device call aborted", "Generic error", "Cancelled by user", "Object ID too low", "Object ID too high", "Object not in heap", "Unknown heap", "Unknown object (invalid DefProc)", "Unknown object (DefProc not in table)", "Message out of range", "Invalid (null) method", "Unknown message", "Manager call not supported", "Bad address", "Network operation in progress", "Network operation timed out", "Connection is busy", "Network attribute not supported", "Network error", "Address in use", "System out of memory", "Connection aborted", "Connection refused", "Not connected", "Already connected", "Connection closed", "Initialization error (interapplication manager)", "Bad occurrence", "Wait on unbound occurrence handler", "Occurrence queue overflow", "Datalog type conflict", "Unused", "Unrecognized type (interapplication manager)", "Memory corrupt", "Failed to make temporary DLL", "Old CIN version", "Drag socket not found", "Failed to load drop-object", "Failed to register OLE object", "Failed to release OLE object", "Format specifier type mismatch", "Unknown format specifier", "Too few format specifiers", "Too many format specifiers", "Scan failed", "Newer CIN version", "Error converting to variant", "Runtime menu error", "Password tampered", "Variant attribute not found", "Incompatible variant data type", "Event data is not available", "Event Store is not present", "Occurrence is not found", "Event Queue is not created", "Event info is not available", "Refnum passed is NULL", "Error retrieving Class GUID", "Error retrieving CoClass GUID", "Error retrieving TypeLib GUID.", "Bad built application magic bytes.", "Specific driver is different from the specific driver associated with the Logical Name.", "There is no session opened to the class driver.", "Max Error", "MAX - Error with config objects", "MAX - Error loading configuration", "MAX - Group not supported"]
        # "Current State"
        # "Do not delete, rename, or modify this frame.\n(this is used to capture unhandled states and typos)"
        # "Handle mistyped state name (developer tool)"
        n136 = Format Into String(format string="Software Exception: Unhandled State \"%s\"." ("message"), error in=w301, w296) -> (resulting string=w304:string, error out=w303:errorcluster)  [unwired: 1 in]
        n137 = call <vilib>:"Error Cluster From Error Code.vi"("show call chain? (False)"=TRUE, "error in (no error)"=w303, "error message (\"\")"=w304, "error code (0)"=w305) -> ("error out"=w302:errorcluster)  [unwired: 5 in]
        n138 = call <vilib>:"Add State(s) to Queue__jki_lib_state_machine.vi"("State(s) in (\"\")"=w300) -> ("States Out"=w299:string)  [unwired: 14 in]
      }
      frame "Initialize Core Data" {
        # "Do not delete, rename, or modify this frame.\n(this is used to determine panel behavior on exit)"
        # "originally closed?"
        # "exe?"
        # "If panel starts closed or is an EXE, then close it when we exit"
        n139 = property class="VI"() -> ("Front Panel.Open"=w314:bool)  [unwired: 2 in, 2 out]
        n140 = property class="App"() -> ("App.Kind"=w313:T8)  [unwired: 2 in, 2 out]
        n141 = control-ref of="Current VI Reference"() -> (w307:refnum<vi>)
        n142 = Not(x=w314) -> (.not. x?=w311:bool)
        n143 = Equal?(x=w313, y=T8."Run Time System" ("Application:Kind")) -> (x = y?=w310:bool)
        n144 = Or(x=w311, y=w310) -> (x .or. y?=w308:bool)
        n145 = Bundle By Name(cluster=w309, "Core.Current VI Reference"=w307, "Core.Close Panel on Exit?"=w308) -> (w316:T12)
        n146 = call <vilib>:"Add State(s) to Queue__jki_lib_state_machine.vi"("State(s) in (\"\")"=w318) -> ("States Out"=w317:string)  [unwired: 14 in]
      }
      frame "Error Handler" {
        # "Unhandled Error -- Display it"
        # "Handle any errors here.\nYou can also output any states to clean-up after errors occur"
        # "Clear error"
        n147 = call <vilib>:"General Error Handler.vi"("error in (no error)"=w320) -> ()  [unwired: 10 in, 5 out]
        n148 = call <vilib>:"Add State(s) to Queue__jki_lib_state_machine.vi"("State(s) in Front (\"\")"="/* Post Error States", "State(s) in (\"\")"=w324) -> ("States Out"=w323:string)  [unwired: 13 in]
      }
      frame "Exit" {
        # "Do not put any code in this frame.\n(No errors that occur here will be handled.)"
        n149 = call <vilib>:"Add State(s) to Queue__jki_lib_state_machine.vi"("State(s) in (\"\")"=w329) -> ("States Out"=w328:string)  [unwired: 14 in]
      }
      frame "---------- Data ----------" {
        # "Do not put any code in this frame.\n(It is a separator no-op. You can make a copy of this frame to create a new Data frame)"
        n150 = call <vilib>:"Add State(s) to Queue__jki_lib_state_machine.vi"("State(s) in (\"\")"=w333) -> ("States Out"=w332:string)  [unwired: 14 in]
      }
      frame "Data: Initialize" {
        w334 = FALSE  # Fire Continues Allowed
        w336 = u32 0  # Tik1
        w335 = u32 0  # Tik2
        w337 = FALSE  # Jet trigger
        w338 = 0.0  # Discharge timing offset
        w339 = 0.0  # Heater timing offset
        w340 = T13 {"Current VI Reference"=refnum, "Close Panel on Exit?"=FALSE}  # Core
        # "Data names and types of shift register data are defined by this bundle."
        # "Initialize the shift-register data, here.\n(data names are defined by what you wire into the bundle function)"
        n151 = Bundle("Core"=w340, "Heater timing offset"=w339, "Discharge timing offset"=w338, "Jet trigger"=w337, "Tik1"=w336, "Tik2"=w335, "Fire Continues Allowed"=w334) -> (w342:T12)  [unwired: 1 in]
        n152 = call <vilib>:"Add State(s) to Queue__jki_lib_state_machine.vi"("State(s) in (\"\")"=w344) -> ("States Out"=w343:string)  [unwired: 14 in]
      }
      frame "Data: Cleanup" {
        # "Cleanup any data and references, here.\n(this is called automatically, by the Macro: Exit)"
        n153 = Unbundle By Name(w345) -> ("Core.Current VI Reference"=w348:refnum<vi>)
        n154 = Close Reference(reference=w348, error in (no error)=w347) -> (error out=w346:errorcluster)
        n155 = call <vilib>:"Add State(s) to Queue__jki_lib_state_machine.vi"("State(s) in (\"\")"=w350) -> ("States Out"=w349:string)  [unwired: 14 in]
      }
      frame "---------- UI ----------" {
        # "Do not put any code in this frame.\n(It is a separator no-op. You can make a copy of this frame to create a new UI frame)"
        n156 = call <vilib>:"Add State(s) to Queue__jki_lib_state_machine.vi"("State(s) in (\"\")"=w354) -> ("States Out"=w353:string)  [unwired: 14 in]
      }
      frame "UI: Initialize" {
        # "Initialize the User Interface, here.\n(this is called automatically, by the Macro: Init)"
        n157 = call <userlib>:"Fit VI window to Largest Dec__ogtk.vi"() -> ()  [unwired: 6 in, 2 out]
        n158 = call <vilib>:"Add State(s) to Queue__jki_lib_state_machine.vi"("State(s) in (\"\")"=w358) -> ("States Out"=w357:string)  [unwired: 14 in]
      }
      frame "UI: Cursor Set" {
        # "Argument"
        # "Set and Unset Cursor Busy.\n(Usage: \"UI: Cursor Set >> Busy|Idle\")"
        n159 = case shown="\"Idle\", Default" w359 {
          tunnel: w361 -> [w366 w368]
          tunnel: [w365 w367] -> w360
          frame "Idle", Default {
            n160 = call <vilib>:"Unset Busy.vi"("error in (no error)"=w366) -> ("error out"=w365:errorcluster)  [unwired: 10 in]
          }
          frame "Busy" {
            n161 = call <vilib>:"Set Busy.vi"("error in (no error)"=w368) -> ("error out"=w367:errorcluster)  [unwired: 9 in, 1 out]
          }
        }
        n162 = call <vilib>:"Add State(s) to Queue__jki_lib_state_machine.vi"("State(s) in (\"\")"=w364) -> ("States Out"=w363:string)  [unwired: 14 in]
      }
      frame "UI: Front Panel State" {
        # "Argument"
        # "Set Front Panel Open or Closed\n(Usage: \"UI: Front Panel State >> Open|Close\")"
        n163 = Unbundle By Name(w371) -> ("Core.Current VI Reference"=w370:refnum<vi>)
        n164 = case shown="\"Close\"" w369 {
          tunnel: w373 -> [w379 w392]
          tunnel: [w381 w393] -> w372
          tunnel: w370 -> [w380 w390]
          frame "Open", Default {
            n165 = property class="VI"(reference=w380, error in=w379) -> (reference out=w377:refnum<vi>, error out=w378:errorcluster, "Front Panel.Open"=w376:bool)
            n166 = case shown="False" w376 {
              tunnel: [w384 w387] -> w381
              tunnel: w378 -> [w383 w387]
              tunnel: w377 -> [w382 _]
              frame False {
                n167 = invoke class="VI" method="FP.Open"(reference=w382, error in=w383, "Activate"=TRUE, "State"=T9."Standard") -> (error out=w384:errorcluster)  [unwired: 1 in, 4 out]
              }
              frame True {
              }
            }
          }
          frame "Close" {
            n168 = property class="VI"(reference=w390, error in=w392) -> (reference out=w389:refnum<vi>, error out=w391:errorcluster, "Front Panel.Open"=w388:bool)
            n169 = case shown="True" w388 {
              tunnel: [w394 w397] -> w393
              tunnel: w391 -> [w394 w396]
              tunnel: w389 -> [_ w395]
              frame False {
              }
              frame True {
                n170 = invoke class="VI" method="FP.Close"(reference=w395, error in=w396) -> (error out=w397:errorcluster)  [unwired: 1 in, 2 out]
              }
            }
          }
        }
        n171 = call <vilib>:"Add State(s) to Queue__jki_lib_state_machine.vi"("State(s) in (\"\")"=w375) -> ("States Out"=w374:string)  [unwired: 14 in]
      }
      frame "---------- Macro ----------" {
        # "Do not put any code in this frame.\n(It is a separator no-op. You can make a copy of this frame to create a new Macro frame)"
        n172 = call <vilib>:"Add State(s) to Queue__jki_lib_state_machine.vi"("State(s) in (\"\")"=w401) -> ("States Out"=w400:string)  [unwired: 14 in]
      }
      frame "Macro: Initialize" {
        w402 = "Data: Initialize\nInitialize Core Data\nUI: Initialize\nUI: Front Panel State >> Open\nCheck if Fire continues allowed\nInitilize Fire Continues\nInit:MegattenuatorStage"  # Data: Initialize Initialize Core Data UI: Initialize UI: Front Panel State >> Open Check if Fire continues allowed Initilize Fire Continues Init:MegattenuatorStage
        # "Initialization Macro\n(This is called once, when the VI starts)"
        n173 = call <vilib>:"Add State(s) to Queue__jki_lib_state_machine.vi"("State(s) in Front (\"\")"=w402, "State(s) in (\"\")"=w406) -> ("States Out"=w405:string)  [unwired: 13 in]
      }
      frame "Macro: Exit" {
        # "Exit Macro\n(This is called once, when the VI exits)"
        n174 = Unbundle By Name(w416) -> ("Core.Close Panel on Exit?"=w415:bool)
        n175 = Release Queue(queue=w408, force destroy? (F)=TRUE) -> (error out=w407:errorcluster)  [unwired: 1 in, 2 out]
        n176 = call <vilib>:"Clear Errors.vi"("error in (no error)"=w407) -> ()  [unwired: 5 in, 2 out]
        n177 = Select(t="UI: Front Panel State >> Close", s=w415, f="") -> (s? t:f=w412:string)
        n178 = call <vilib>:"Add State(s) to Queue__jki_lib_state_machine.vi"("State(s) in (\"\")"=w412, "State(s) at Back (\"\")"="Data: Cleanup\nExit") -> ("States Out"=w410:string)  [unwired: 13 in]
        n179 = call <vilib>:"Add State(s) to Queue__jki_lib_state_machine.vi"("State(s) in Front (\"\")"=w410, "State(s) in (\"\")"=w419) -> ("States Out"=w418:string)  [unwired: 13 in]
      }
      frame "---------- New Category ----------" {
        # "Template Separator\n(You can make a copy of, or modify, this frame)"
        n180 = call <vilib>:"Add State(s) to Queue__jki_lib_state_machine.vi"("State(s) in (\"\")"=w423) -> ("States Out"=w422:string)  [unwired: 14 in]
      }
      frame "Check Megattenuator Stage Status" {
        n181 = property on="Position.Ch1::44" class="DigNum (strict)"() -> ("Value"=w424:dbl)  [unwired: 2 in, 2 out]
        n182 = case shown="0, 1" w424 {
          tunnel: ["IN" "Unknown/Moving" "OUT"] -> w425
          frame 0, 1 {
            n183 = property on="MoveStage" class="Bool (strict)"("Value"=TRUE) -> ()  [unwired: 2 in, 2 out]
          }
          frame 2, Default {
          }
          frame 149..151 {
            n184 = property on="MoveStage" class="Bool (strict)"("Value"=FALSE) -> ()  [unwired: 2 in, 2 out]
          }
        }
        n185 = property on="CurrentStatus" class="Str"("Value"=w425) -> ()  [unwired: 2 in, 2 out]
        n186 = call <vilib>:"Add State(s) to Queue__jki_lib_state_machine.vi"("State(s) in (\"\")"=w429) -> ("States Out"=w428:string)  [unwired: 14 in]
      }
      frame "Init:MegattenuatorStage" {
        # "Template Separator\n(You can make a copy of, or modify, this frame)"
        n187 = disable-structure shown="Disabled" {
          frame Disabled {
            n188 = flat-sequence {
              frame #0 {
                n189 = call <vilib>:"Set Busy.vi"("disable click? (T)"=TRUE, "cursor ID"=refnum<k1> refnum) -> ()  [unwired: 8 in, 2 out]
              }
              frame #1 {
                n190 = while {
                  tunnel: [w450] -> w442
                  i -> [w445]
                  stop <- w446 stop-if-true
                  n191 = property on="Position.Ch1::44" class="DigNum (strict)"() -> ("Value"=w450:dbl)  [unwired: 2 in, 2 out]
                  n192 = Equal?(x=50, y=w445) -> (x = y?=w443:bool)
                  n193 = Not Equal?(x=w450, y=0.0) -> (x != y?=w447:bool)
                  n194 = Wait (ms)(milliseconds to wait=u32 100) -> ()  [unwired: 1 out]
                  n195 = Or(x=w447, y=w443) -> (x .or. y?=w446:bool)
                }
                n196 = case shown="0, 1" w442 {
                  tunnel: ["IN" "Unknown" "OUT"] -> w441
                  frame 0, 1 {
                    n197 = property on="MoveStage" class="Bool (strict)"("Value"=TRUE) -> ()  [unwired: 2 in, 2 out]
                  }
                  frame 2, Default {
                    n198 = property on="MoveStage" class="Bool (strict)"("DisabledEnum"=T7."Disabled" ("Disabled")) -> ()  [unwired: 2 in, 2 out]
                  }
                  frame 149..151 {
                    n199 = property on="MoveStage" class="Bool (strict)"("Value"=FALSE) -> ()  [unwired: 2 in, 2 out]
                  }
                }
                n200 = property on="CurrentStatus" class="Str"("Value"=w441) -> ()  [unwired: 2 in, 2 out]
              }
              frame #2 {
                n201 = call <vilib>:"Unset Busy.vi"() -> ()  [unwired: 11 in, 1 out]
              }
            }
          }
          frame Enabled {
          }
        }
        n202 = call <vilib>:"Add State(s) to Queue__jki_lib_state_machine.vi"("State(s) in (\"\")"=w438) -> ("States Out"=w437:string)  [unwired: 14 in]
      }
      frame "CheckTimeFire" {
        # "Your code here.\n(You can make a copy of, or modify, this frame)"
        n203 = Unbundle By Name(w463) -> ("Tik1"=w468:u32)
        n204 = Tick Count (ms)() -> (millisecond timer value=w470:u32)
        n205 = Unbundle By Name(w463) -> ("Fire Continues Allowed"=w460:bool)
        n206 = Reciprocal(x="Rate (Hz)") -> (1/x=w459:dbl)
        n207 = Subtract(x=w470, y=w468) -> (x-y=w471:u32)
        n208 = Multiply(x=1000.0, y=w459) -> (x*y=w458:dbl)
        n209 = Greater?(x=w471, y=w458) -> (0:w466:bool)
        n210 = And(x=w466, y="value0::22") -> (x .and. y?=w462:bool)
        n211 = And(x=w460, y=w462) -> (x .and. y?=w461:bool)
        n212 = case shown="True" w461 {
          tunnel: w470 -> [_ w478]
          tunnel: [w476 w478] -> w469
          tunnel: w468 -> [w476 _]
          tunnel: [_ "Action: Fire" ("State(s) in Front (\"\")")] -> w465
          frame False {
          }
          frame True {
          }
        }
        n213 = Bundle By Name(cluster=w463, "Tik1"=w469) -> (w472:T12)
        n214 = call <vilib>:"Add State(s) to Queue__jki_lib_state_machine.vi"("State(s) in Front (\"\")"=w465, "State(s) in (\"\")"=w475) -> ("States Out"=w474:string)  [unwired: 13 in]
        "Fire continues Indicator" <- "value0::22"
      }
      frame "Initilize Fire Continues" {
        # "Your code here.\n(You can make a copy of, or modify, this frame)"
        n215 = Unbundle By Name(w482) -> ("Fire Continues Allowed"=w481:bool)
        n216 = property on="value0::22" class="Bool (strict)"(error in=w484, "Visible"=w481) -> (error out=w483:errorcluster)  [unwired: 1 in, 1 out]
        n217 = Not(x=w481) -> (.not. x?=w479:bool)
        n218 = property on="Fire continues Indicator" class="Bool (strict)"(error in=w483, "Visible"=w479) -> (error out=w480:errorcluster)  [unwired: 1 in, 1 out]
        n219 = call <vilib>:"Add State(s) to Queue__jki_lib_state_machine.vi"("State(s) in (\"\")"=w486) -> ("States Out"=w485:string)  [unwired: 14 in]
      }
      frame "Check if Fire continues allowed" {
        # "Check if it is allowed computer"
        # "Your code here.\n(You can make a copy of, or modify, this frame)"
        n220 = String To IP() -> (0:w494:u32)  [unwired: 1 in]
        n221 = IP To String(1:TRUE ("dot notation? (F)"), 2:w494) -> (0:w495:string)
        n222 = Equal?(x=w495, y="192.168.14.2") -> (x = y?=w489:bool)
        n223 = Not(x=w489) -> (.not. x?=w490:bool)
        n224 = Bundle By Name(cluster=w492, "Fire Continues Allowed"=w489) -> (w491:T12)
        n225 = property on="Allow Fire Continues" class="Bool (strict)"(error in=w488, "Visible"=w490) -> (error out=w487:errorcluster)  [unwired: 1 in, 1 out]
        n226 = call <vilib>:"Add State(s) to Queue__jki_lib_state_machine.vi"("State(s) in (\"\")"=w498) -> ("States Out"=w497:string)  [unwired: 14 in]
      }
      frame "CheckTime2" {
        # "Your code here.\n(You can make a copy of, or modify, this frame)"
        n227 = Unbundle By Name(w507) -> ("Tik2"=w500:u32)
        n228 = Tick Count (ms)() -> (millisecond timer value=w502:u32)
        n229 = Subtract(x=w502, y=w500) -> (x-y=w505:u32)
        n230 = Greater?(x=w505, y=5000) -> (0:w503:bool)
        n231 = case shown="True" w503 {
          tunnel: w502 -> [_ w513]
          tunnel: [w511 w513] -> w501
          tunnel: w500 -> [w511 _]
          tunnel: [_ "Action: update expt vars\nAction: save screenshot"] -> w499
          frame False {
          }
          frame True {
          }
        }
        n232 = Bundle By Name(cluster=w507, "Tik2"=w501) -> (w506:T12)
        n233 = call <vilib>:"Add State(s) to Queue__jki_lib_state_machine.vi"("State(s) in Front (\"\")"=w499, "State(s) in (\"\")"=w510) -> ("States Out"=w509:string)  [unwired: 13 in]
      }
      frame "Action: Fire" {
        n234 = call <vilib>:"Add State(s) to Queue__jki_lib_state_machine.vi"("State(s) in (\"\")"=w517) -> ("States Out"=w516:string)  [unwired: 14 in]
      }
      frame "Action: Move SMF" {
        n235 = call <vilib>:"Add State(s) to Queue__jki_lib_state_machine.vi"("State(s) in (\"\")"=w521) -> ("States Out"=w520:string)  [unwired: 14 in]
      }
      frame "Action: Move DPM" {
        # "Debris"
        # "z"
        # "y"
        n236 = Add(x="Position.Stage C::11", y="DPM intercept") -> (x+y=w531:dbl)
        n237 = Subtract(x="Position.Stage B::12", y=w531) -> (x-y=w530:dbl)
        n238 = Absolute Value(x=w530) -> (abs(x)=w529:dbl)
        n239 = Less?(x=w529, y=3.0) -> (x < y?=w528:bool)
        n240 = case shown="True" w528 {
          tunnel: w525 -> [w535 w545]
          tunnel: [w535 w546] -> w524
          tunnel: "Position.Stage B::12" -> [_ w543]
          tunnel: "Position.Stage C::11" -> [_ w542]
          frame False {
          }
          frame True {
            w538 = 5.0 ("y")
            n241 = Negate(x=w538) -> (-x=w537:dbl)
            n242 = Select(t=w538, s="DPM Direction", f=w537) -> (s? t:f=w536:dbl)
            n243 = Add(x=w536, y=w542) -> (x+y=w541:dbl)
            n244 = Add(x=w543, y=w536) -> (x+y=w540:dbl)
            n245 = property on="Position.Stage C::11" class="DigNum (strict)"(error in=w545, "Val(Sgnl)"=w541) -> (error out=w544:errorcluster)  [unwired: 1 in, 1 out]
            n246 = property on="Position.Stage B::12" class="DigNum (strict)"(error in=w544, "Val(Sgnl)"=w540) -> (error out=w546:errorcluster)  [unwired: 1 in, 1 out]
          }
        }
        n247 = call <vilib>:"Add State(s) to Queue__jki_lib_state_machine.vi"("State(s) in (\"\")"=w534) -> ("States Out"=w533:string)  [unwired: 14 in]
      }
      frame "Action: update expt vars" {
        # "Your code here.\n(You can make a copy of, or modify, this frame)"
        n248 = call <vilib>:"Add State(s) to Queue__jki_lib_state_machine.vi"("State(s) in (\"\")"=w550) -> ("States Out"=w549:string)  [unwired: 14 in]
      }
      frame "Action: SendScanParameters" {
        # "Your code here.\n(You can make a copy of, or modify, this frame)"
        n249 = call "BELLA PW scan mode shot control shutter.vi"("PostScanRate"="value6::42", "ScanShotControl"="value0::43") -> ("error out"=w551:errorcluster, "delay D to set"=w552:dbl)  [unwired: 8 in]
        n250 = property on="Delay.Ch D::10" class="DigNum (strict)"("Val(Sgnl)"=w552) -> ()  [unwired: 2 in, 2 out]
        n251 = flat-sequence {
          tunnel: w551 -> [_]
          frame #0 {
            n252 = call "TimeoutDialog.vi"("message 2"="expt editor set up" ("message"), "Timeout(ms)"=u32 1000) -> ()  [unwired: 9 in]
          }
        }
        n253 = call <vilib>:"Add State(s) to Queue__jki_lib_state_machine.vi"("State(s) in (\"\")"=w558) -> ("States Out"=w557:string)  [unwired: 14 in]
      }
      frame "Action: save screenshot" {
        # "Your code here.\n(You can make a copy of, or modify, this frame)"
        n254 = case shown="True" "Save \ncreenshots" {
          frame False {
          }
          frame True {
            n255 = invoke class="VI" method="FP.Get Image"() -> ("image data"=w568:T10)  [unwired: 6 in, 5 out]
            n256 = call <vilib>:"Write PNG File.vi"("image data"=w568, "path to PNG file"=path "N:/data/ECS dumps/Logmaker Screenshot/frontpanel.png" ("report file path")) -> ("error out"=→"error out":errorcluster)  [unwired: 8 in, 1 out]
          }
        }
        n257 = call <vilib>:"Add State(s) to Queue__jki_lib_state_machine.vi"("State(s) in (\"\")"=w565) -> ("States Out"=w564:string)  [unwired: 14 in]
      }
    }
  }
  n258 = for {
    N: 25 -> [_]
    tunnel: w4 -> [w571]
    tunnel: [w571] -> w3
    tunnel: [w569] -> w1
    stop <- w569 stop-if-true
    n259 = local read "got manpar ofi data"() -> (w573:bool)
    n260 = local read "got manpar ofi bool data"() -> (w572:bool)
    n261 = Wait (ms)(milliseconds to wait=u32 1000) -> ()  [unwired: 1 out]
    n262 = And(x=w573, y=w572) -> (x .and. y?=w569:bool)
  }
  n263 = disable-structure shown="Disabled" {
    frame Disabled {
    }
    frame Enabled {
    }
  }
  n264 = case shown="True" w1 {
    tunnel: w3 -> [_ w574]
    frame False {
    }
    frame True {
      n265 = call <userlib>:"Wait (ms)__ogtk.vi"("error in (no error)"=w574, "milliseconds to wait"=u32 3000) -> ("error out"=w576:errorcluster)  [unwired: 8 in, 1 out]
      n266 = property on="set expt editor" class="Bool (strict)"(error in=w576, "Val(Sgnl)"=TRUE ("Value (Signaling)")) -> ()  [unwired: 1 in, 2 out]
    }
  }
  n267 = disable-structure shown="Disabled" {
    frame Disabled {
    }
    frame Enabled {
    }
  }
  n268 = disable-structure shown="Disabled" {
    frame Disabled {
      n269 = call "get set udp value from dev var alias array.vi"() -> ()  [unwired: 9 in, 3 out]
    }
    frame Enabled {
    }
  }
  "CurrentStatus" <- ""
